vi "Actuate Digital Line.vi"(8 "error in":errorcluster, 9 "timeout":dbl=10.0 format="%0.2f", 10 "state":bool, 11 "DO-Line Ref":refnum<k21>) -> (0 "error out":errorcluster, 3 "DO-Line Ref out":refnum<k21>)   [LabVIEW 2017]
doc: "Developed by Kevin Thompson\nThompson Engineering, LLC\nkevin@thompsonengineering.net"
uses:
  <vilib>/DAQmx/write.llb/DAQmx Write (Digital Bool 1Line 1Point).vi
  <vilib>/DAQmx/miscellaneous.llb/DAQmx Fill In Error Info.vi
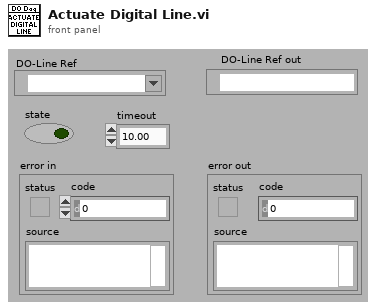
[diagram p1: front panel]
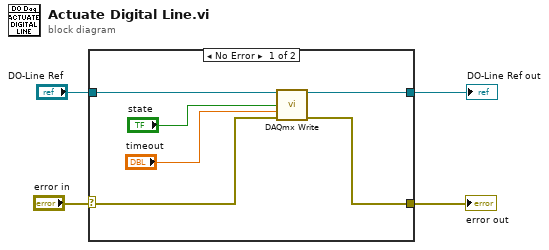
[diagram p0: block diagram]
diagram:
  n1 = case shown="No Error" "error in" {
    selector: "error in" -> [w5 w11]
    tunnel: "DO-Line Ref" -> [w10 w12]
    tunnel: [w9 w12] -> w3
    tunnel: [w8 w11] -> w2
    frame No Error {
      n2 = call-poly <vilib>:"DAQmx Write.vi"("task/channels in"=w10, "data"="state", "timeout"="timeout", "error in"=w5) -> ("task out"=w9:refnum<k21>, "error out"=w8:errorcluster)  [unwired: 9 in, 1 out]
    }
    frame Error {
    }
  }
  "error out" <- w2
  "DO-Line Ref out" <- w3
